vi "i32 to dec string small.vi"(7 "number":i32) -> (8 "String":string)   [LabVIEW 2018]
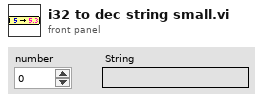
[diagram p1: front panel]
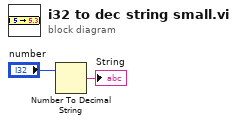
[diagram p0: block diagram]
diagram:
  n1 = Number To Decimal String(number="number") -> (decimal integer string=→"String":string)  [unwired: 1 in]
